vi "fft_norm_test.vi"() -> ()   [LabVIEW 2014]
uses:
  <vilib>/Analysis/2dsp.llb/Inverse Real FFT.vi
  <vilib>/Analysis/2dsp.llb/Real FFT.vi
  <vilib>/Analysis/NI_AALPro.lvlib
panel:
  out "FFT":cdb
  in  "Size":i32=256
  in  "Magnitude":cdb=1.0+0.0i
  in  "Channel":i32=5
  out "Waveform Graph":dbl[](graph)
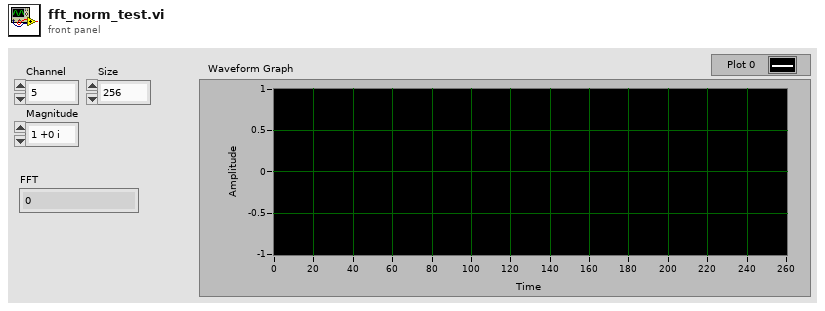
[diagram p1: front panel]
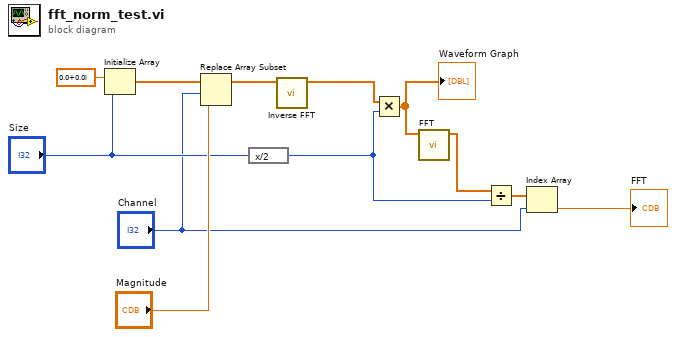
[diagram p0: block diagram]
diagram:
  n1 = Initialize Array(cdb 0.0+0.0i ("element"), "Size") -> (w11:cdb[])
  n2 = Replace Array Subset(array=w11, new element="Magnitude", index="Channel") -> (w9:cdb[])
  n3 = expression code="x/2"("Size") -> (w2:i32)
  n4 = call-poly <vilib>:"Inverse FFT.vi"("FFT {X}"=w9) -> ("X"=w8:dbl[])  [unwired: 9 in, 1 out]
  n5 = Multiply(x=w8, y=w2) -> (x*y=w6:dbl[])
  "Waveform Graph" <- w6
  n6 = call-poly <vilib>:"FFT.vi"("X"=w6) -> ("FFT {X}"=w3:cdb[])  [unwired: 9 in, 1 out]
  n7 = Divide(x=w3, y=w2) -> (x/y=w1:cdb[])
  n8 = Index Array(array=w1, index="Channel") -> (element=→"FFT":cdb)
